vi "Draw Raw.vi"(8 "error in (no error)":errorcluster, 11 "Shape in":refnum<class "Shape.lvclass">) -> (0 "error out":errorcluster, 2 "Raw":string, 3 "Shape out":refnum<class "Shape.lvclass">)   [LabVIEW 2017, in "LV Image Editor Framework.lvlib" / "Shape.lvclass"]
uses:
  Shape.lvclass
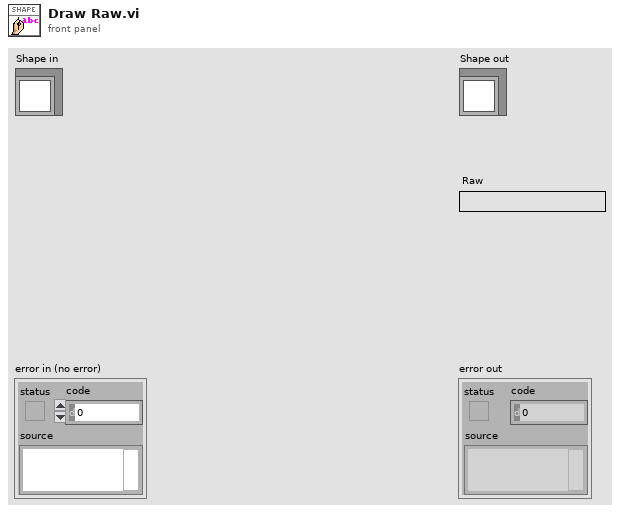
[diagram p1: front panel]
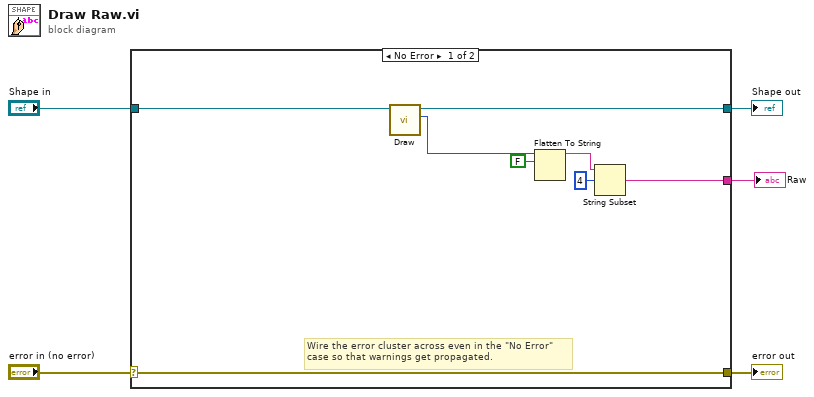
[diagram p0: block diagram]
diagram:
  n1 = case shown="No Error" "error in (no error)" {
    selector: "error in (no error)" -> [w13 w15]
    tunnel: [w13 w15] -> w4
    tunnel: [w11 w14] -> w2
    tunnel: "Shape in" -> [w12 w14]
    tunnel: [w6 _] -> w1
    frame No Error {
      # "Wire the error cluster across even in the \"No Error\"\ncase so that warnings get propagated."
      n2 = call-dynamic "Draw.vi"("Shape in"=w12) -> ("Picture"=w10:picture, "Shape out"=w11:refnum<class "Shape.lvclass">)  [unwired: 8 in, 1 out]
      n3 = Flatten To String(anything=w10, prepend array or string size? (T)=FALSE) -> (data string=w9:string)  [unwired: 2 in, 2 out]
      n4 = String Subset(string=w9, offset (0)=4) -> (substring=w6:string)  [unwired: 1 in]
    }
    frame Error {
    }
  }
  "error out" <- w4
  "Shape out" <- w2
  "Raw" <- w1
